vi "Init YZ 2D.vi"(6 "error in":T2, 7 "Z-Axis Communications Config":T1={"GPIB address"=22, "GPIB bus"=0, "connection ID"=refnum, "IP"="192.168.2.200", "Active Comm Interface"=0, "Serial Port"="", "Programmer Type"=0} {"Programmer Type" items=["Model 430", "Model 420"]; "Active Comm Interface" items=["TCP/IP (Model 430 Only)", "RS232", "IEEE488"]}, 9 "Y-Axis Communications Config":T1={"GPIB address"=22, "GPIB bus"=0, "connection ID"=refnum, "IP"="192.168.2.200", "Active Comm Interface"=0, "Serial Port"="", "Programmer Type"=0} {"Programmer Type" items=["Model 430", "Model 420"]; "Active Comm Interface" items=["TCP/IP (Model 430 Only)", "RS232", "IEEE488"]}) -> (2 "error out":T2)   [LabVIEW 2018]
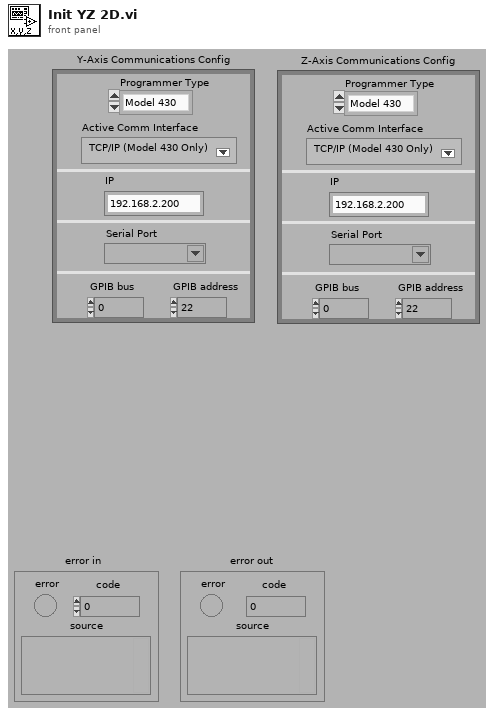
[diagram p1: front panel]
types:
  T1 = cluster{"GPIB address":i16, "GPIB bus":i16, "connection ID":refnum<k5>, "IP":string, "Active Comm Interface":u16, "Serial Port":refnum<visa-resource-name>, "Programmer Type":u16}
  T2 = cluster{"error":bool, "code":i32, "source":string}
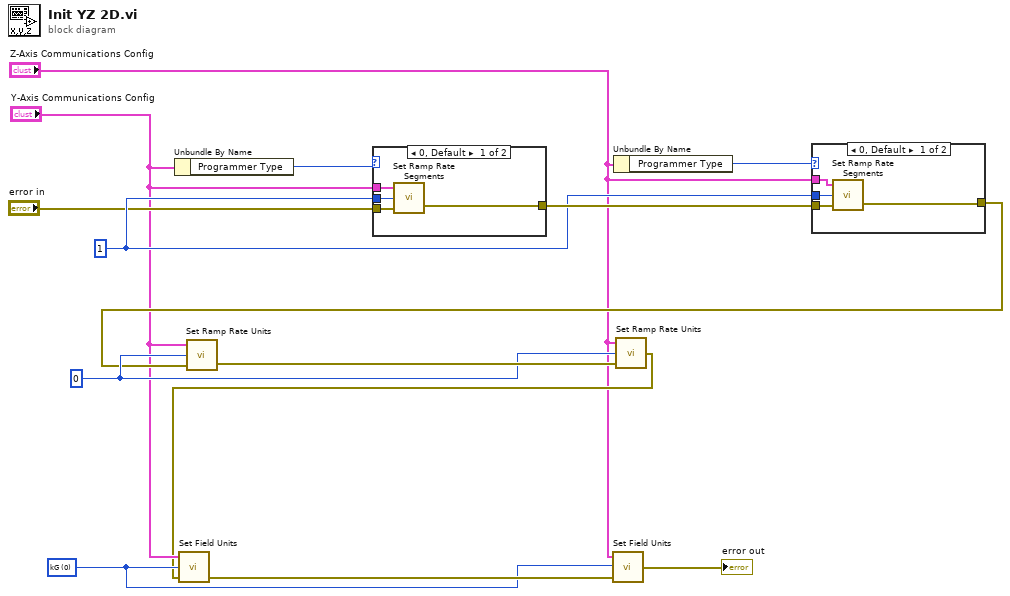
[diagram p0: block diagram]
diagram:
  w9 = 0
  w11 = 1
  w8 = u16 0 items=["kG", "Tesla"] ("Field Units")
  n1 = Unbundle By Name("Y-Axis Communications Config") -> ("Programmer Type"=w4:u16)
  n2 = case shown="0, Default" w4 {
    tunnel: w11 -> [w18 _]
    tunnel: "error in" -> [w17 w19]
    tunnel: [w16 w19] -> w12
    tunnel: "Y-Axis Communications Config" -> [w15 _]
    frame 0, Default {
      n3 = call "Set Ramp Rate Segments.vi"("error in"=w17, "Segments"=w18, "Communications Config"=w15) -> ("error out"=w16:T2)
    }
    frame 1 {
    }
  }
  n4 = Unbundle By Name("Z-Axis Communications Config") -> ("Programmer Type"=w3:u16)
  n5 = case shown="0, Default" w3 {
    tunnel: w11 -> [w23 _]
    tunnel: w12 -> [w22 w24]
    tunnel: [w21 w24] -> w6
    tunnel: "Z-Axis Communications Config" -> [w20 _]
    frame 0, Default {
      n6 = call "Set Ramp Rate Segments.vi"("error in"=w22, "Segments"=w23, "Communications Config"=w20) -> ("error out"=w21:T2)
    }
    frame 1 {
    }
  }
  n7 = call "Set Ramp Rate Units.vi"("error in"=w6, "Ramp Rate Units"=w9, "Communications Config"="Y-Axis Communications Config") -> ("error out"=w10:T2)
  n8 = call "Set Ramp Rate Units.vi"("error in"=w10, "Ramp Rate Units"=w9, "Communications Config"="Z-Axis Communications Config") -> ("error out"=w2:T2)
  n9 = call "Set Field Units.vi"("error in"=w2, "Field Units"=w8, "Communications Config"="Y-Axis Communications Config") -> ("error out"=w14:T2)
  n10 = call "Set Field Units.vi"("error in"=w14, "Field Units"=w8, "Communications Config"="Z-Axis Communications Config") -> ("error out"=→"error out":T2)
